vi "Set Impedance Analog.vi"(3 "error in":errorcluster, 4 "p1":i8, 5 "COM Port in":refnum<visa-resource-name>) -> (0 "error out":errorcluster, 1 "OK":bool, 2 "COM Port out":refnum<visa-resource-name>)   [LabVIEW 2013]
doc: "This command selects the input impedance and voltage range for the analog modulation\ninput.\n\nValid values for the parameter “p1” are:\n“1”: input voltage range 0..5V, impedance 1.2kOhm\n“0”: input voltage range 0..1V, impedance 50Ohm\n\nAll other values will be refused."
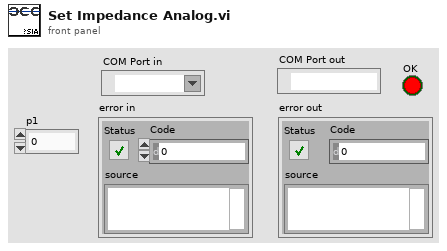
[diagram p1: front panel]
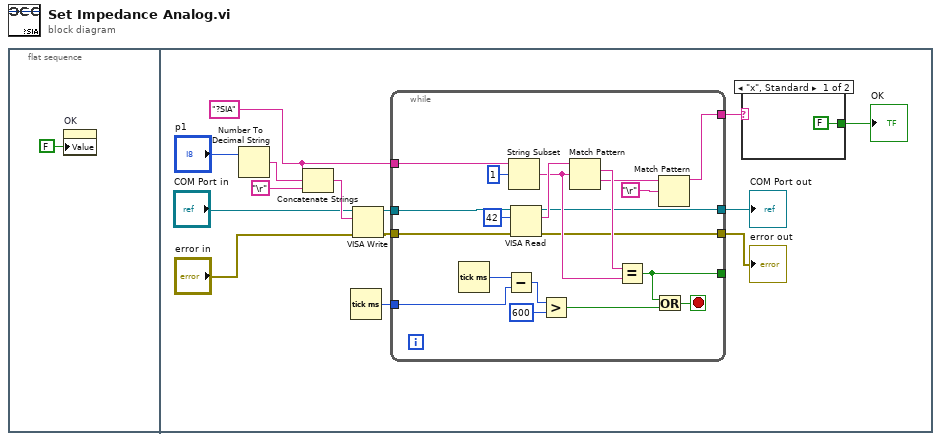
[diagram p0: block diagram]
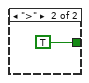
[diagram p2: hidden frame]
diagram:
  n1 = flat-sequence {
    frame #0 {
      n2 = property on="OK" class="Bool. (strikt)"("Value"=FALSE ("OK")) -> ()  [unwired: 2 in, 2 out]
    }
    frame #1 {
      w8 = "?SIA" ("Schreibpuffer")
      n3 = Number To Decimal String(number="p1") -> (decimal integer string=w2:string)  [unwired: 1 in]
      n4 = Concatenate Strings(w8, w2, "\r") -> (w13:string)
      n5 = Tick Count (ms)() -> (millisecond timer value=w7:u32)
      n6 = VISA Write(VISA resource name="COM Port in", write buffer=w13, error in (no error)="error in") -> (VISA resource name out=w10:refnum<visa-resource-name>, error out=w9:errorcluster)  [unwired: 1 out]
      n7 = while {
        tunnel: [w32] -> w15
        tunnel: [w31] -> w14
        tunnel: [w30] -> w6
        tunnel: [w26] -> _
        tunnel: w10 -> [w19]
        tunnel: w9 -> [w28]
        tunnel: w8 -> [w27]
        tunnel: w7 -> [w23]
        stop <- w25 stop-if-true
        n8 = Tick Count (ms)() -> (millisecond timer value=w24:u32)
        n9 = Subtract(x=w24, y=w23) -> (x-y=w22:u32)
        n10 = String Subset(string=w27, offset (0)=1 ("Offset (0)")) -> (substring=w33:string)  [unwired: 1 in]
        n11 = VISA Read(VISA resource name=w19, byte count=u32 42 ("Byte-Anzahl"), error in (no error)=w28) -> (VISA resource name out=w32:refnum<visa-resource-name>, read buffer=w36:string, error out=w31:errorcluster)  [unwired: 1 out]
        n12 = Greater?(x=w22, y=u32 600) -> (0:w20:bool)
        n13 = Match Pattern(string=w36, regular expression=w33) -> (match substring=w35:string, after substring=w29:string)  [unwired: 1 in, 2 out]
        n14 = Equal?(x=w35, y=w33) -> (x = y?=w26:bool)
        n15 = Or(x=w26, y=w20) -> (x .or. y?=w25:bool)
        n16 = Match Pattern(string=w29, regular expression="\r") -> (before substring=w30:string)  [unwired: 1 in, 3 out]
      }
      "COM Port out" <- w15
      "error out" <- w14
      n17 = case shown="\"x\", Standard" w6 {
        tunnel: [FALSE TRUE] -> w5
        frame "x", Default {
        }
        frame ">" {
        }
      }
      "OK" <- w5
    }
  }
